vi "sub vi - analog 1st setup v2.vi"() -> (10 "loop time":dbl format="%.6g", 15 "error out":errorcluster)   [LabVIEW 2013]
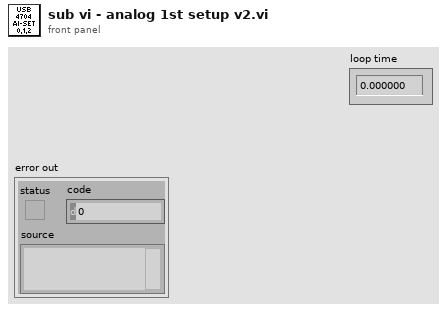
[diagram p1: front panel]
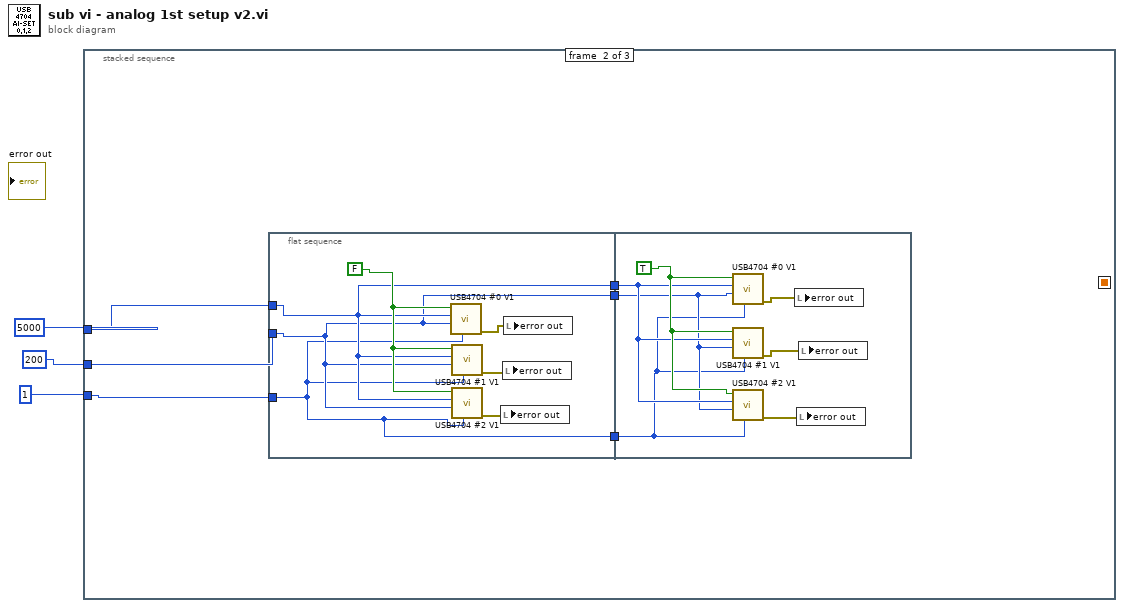
[diagram p0: block diagram]
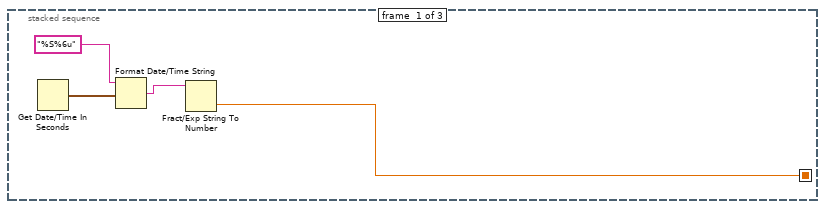
[diagram p2: hidden frame]
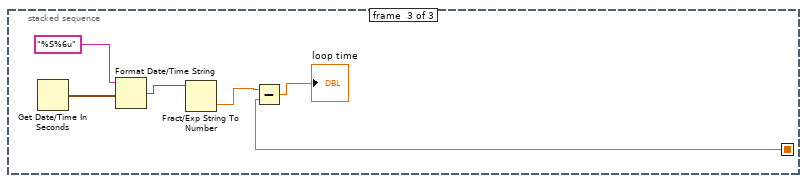
[diagram p3: hidden frame]
diagram:
  n1 = stacked-sequence {
    seq-local: [w4 _ _] -> [_ _ w29]
    tunnel: 1 -> [_ w11 _]
    tunnel: 5000 -> [_ w13 _]
    tunnel: 200 -> [_ w12 _]
    frame #0 {
      n2 = Get Date/Time In Seconds() -> (seconds since 1Jan1904=w6:timestamp)
      n3 = Format Date/Time String(time format string (%c)="%S%6u", seconds (now)=w6) -> (date/time string=w5:string)  [unwired: 1 in]
      n4 = Fract/Exp String To Number(string=w5) -> (number=w4:dbl)  [unwired: 3 in, 1 out]
    }
    frame #1 {
      n5 = flat-sequence {
        tunnel: w13 -> [w19]
        tunnel: w12 -> [w18]
        tunnel: w11 -> [w17]
        tunnel: [w19] -> w10
        tunnel: [w18] -> w9
        tunnel: [w17] -> w8
        tunnel: w10 -> [w26]
        tunnel: w9 -> [w25]
        tunnel: w8 -> [w24]
        frame #0 {
          w20 = FALSE
          n6 = call "USB4704 #0 V1.vi"("Time out"=w17, "Samples"=w18, "Rate"=w19, "start/stop"=w20) -> ("error out"=w16:errorcluster)  [unwired: 6 in, 1 out]
          n7 = call "USB4704 #1 V1.vi"("TimeOut"=w17, "Cycles"=w18, "Rate"=w19, "Start/Stop"=w20) -> ("error out"=w15:errorcluster)  [unwired: 6 in, 1 out]
          n8 = call "USB4704 #2 V1.vi"("TimeOut"=w17, "Cycles"=w18, "Rate"=w19, "Start/Stop"=w20) -> ("error out"=w14:errorcluster)  [unwired: 6 in, 1 out]
          n9 = local write "error out"(w14) -> ()
          n10 = local write "error out"(w15) -> ()
          n11 = local write "error out"(w16) -> ()
        }
        frame #1 {
          w27 = TRUE
          n12 = call "USB4704 #0 V1.vi"("Time out"=w24, "Samples"=w25, "Rate"=w26, "start/stop"=w27) -> ("error out"=w23:errorcluster)  [unwired: 6 in, 1 out]
          n13 = call "USB4704 #1 V1.vi"("TimeOut"=w24, "Cycles"=w25, "Rate"=w26, "Start/Stop"=w27) -> ("error out"=w22:errorcluster)  [unwired: 6 in, 1 out]
          n14 = call "USB4704 #2 V1.vi"("TimeOut"=w24, "Cycles"=w25, "Rate"=w26, "Start/Stop"=w27) -> ("error out"=w21:errorcluster)  [unwired: 6 in, 1 out]
          n15 = local write "error out"(w23) -> ()
          n16 = local write "error out"(w21) -> ()
          n17 = local write "error out"(w22) -> ()
        }
      }
    }
    frame #2 {
      n18 = Get Date/Time In Seconds() -> (seconds since 1Jan1904=w32:timestamp)
      n19 = Format Date/Time String(time format string (%c)="%S%6u", seconds (now)=w32) -> (date/time string=w31:string)  [unwired: 1 in]
      n20 = Fract/Exp String To Number(string=w31) -> (number=w30:dbl)  [unwired: 3 in, 1 out]
      n21 = Subtract(x=w30, y=w29) -> (x-y=→"loop time":dbl)
    }
  }
